vi "_PC_Spectrafilter calc_noise_feature.vi"(8 "error in (no error)":errorcluster, 10 "noise range":cluster{"start":dbl, "end":dbl}, 11 "spectrum data":cluster{"X":dbl[], "Y":sgl[]}) -> (0 "error out":errorcluster, 2 "noise feature":cluster{"noise diff":sgl, "median":dbl})   [LabVIEW 2018]
uses:
  <vilib>/Analysis/NI_AALBase.lvlib
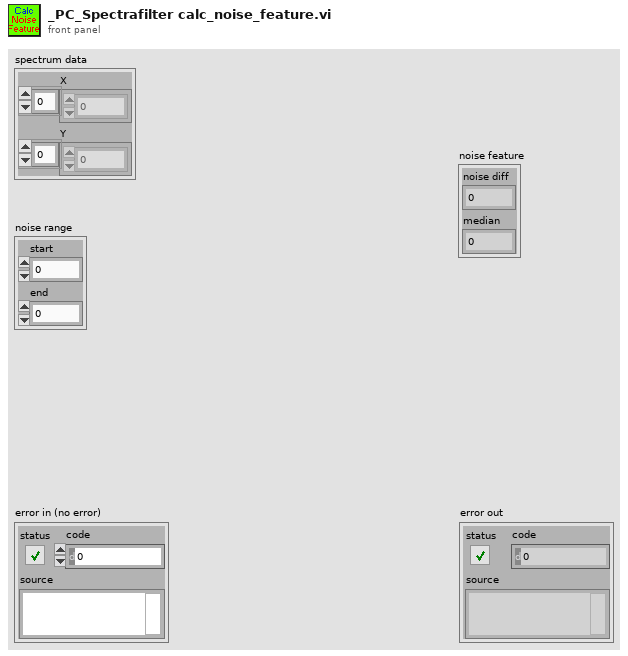
[diagram p1: front panel]
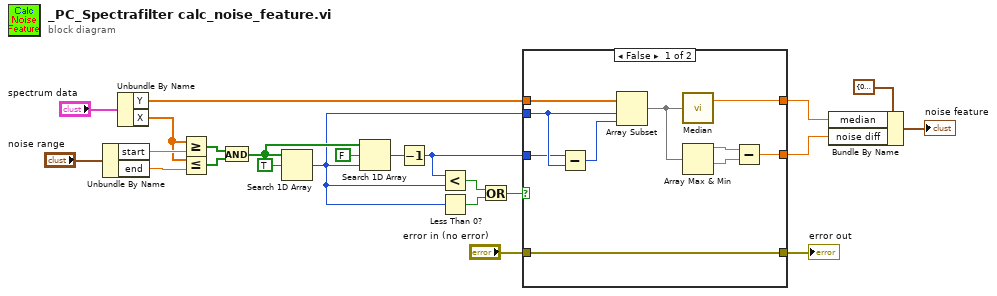
[diagram p0: block diagram]
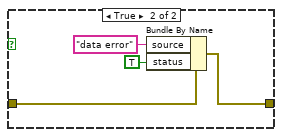
[diagram p2: hidden frame]
diagram:
  n1 = Unbundle By Name("noise range") -> ("start"=w15:dbl, "end"=w14:dbl)
  n2 = Unbundle By Name("spectrum data") -> ("Y"=w12:sgl[], "X"=w13:dbl[])
  n3 = Greater Or Equal?(x=w13, y=w15) -> (x >= y?=w23:bool[])
  n4 = Less Or Equal?(x=w13, y=w14) -> (x <= y?=w22:bool[])
  n5 = And(x=w23, y=w22) -> (x .and. y?=w20:bool[])
  n6 = Search 1D Array(1D array=w20, element=TRUE) -> (index of element=w7:i32)  [unwired: 1 in]
  n7 = Search 1D Array(1D array=w20, element=FALSE, start index (0)=w7) -> (index of element=w18:i32)
  n8 = Decrement(x=w18) -> (x-1=w8:i32)
  n9 = Less?(x=w8, y=w7) -> (x < y?=w11:bool)
  n10 = Less Than 0?(x=w7) -> (x < 0?=w10:bool)
  n11 = Or(x=w11, y=w10) -> (x .or. y?=w9:bool)
  n12 = case shown="False" w9 {
    tunnel: w12 -> [w33 _]
    tunnel: w8 -> [w24 _]
    tunnel: w7 -> [w25 _]
    tunnel: [w31 _] -> w3
    tunnel: [w27 _] -> w2
    tunnel: "error in (no error)" -> [w26 w35]
    tunnel: [w26 w34] -> w5
    frame False {
      n13 = Subtract(x=w24, y=w25) -> (x-y=w32:i32)
      n14 = Array Subset(array=w33, index=w25, length=w32) -> (w30:sgl[])
      n15 = call <vilib>:"Median.vi"("X"=w30) -> ("median"=w31:dbl)  [unwired: 1 out]
      n16 = Array Max & Min(array=w30) -> (max value=w29:sgl, min value=w28:sgl)  [unwired: 2 out]
      n17 = Subtract(x=w29, y=w28) -> (x-y=w27:sgl)
    }
    frame True {
      n18 = Bundle By Name(cluster=w35, "source"="data error", "status"=TRUE) -> (w34:errorcluster)
    }
  }
  "error out" <- w5
  n19 = Bundle By Name(cluster=cluster{"noise diff":sgl, "median":dbl} {"noise diff"=0.0, "median"=0.0} ("noise feature"), "median"=w3, "noise diff"=w2) -> (→"noise feature":cluster{"noise diff":sgl, "median":dbl})
